vi "visa write read buffer.vi"() -> ()   [LabVIEW 2010]
doc: "This VI will write commands and reads responses from a VISA device."
panel:
  in  "Send Message":bool
  in  "VISA resource name":refnum<visa-resource-name>
  out "Read Buffer":string
  in  "Write Buffer":string="MEAS:AC?"
  in  "stop":bool
  # "Enter message in the Write Buffer\ncontrol and click Send Message to\nsend the message and read the \nresponse from the instrument."
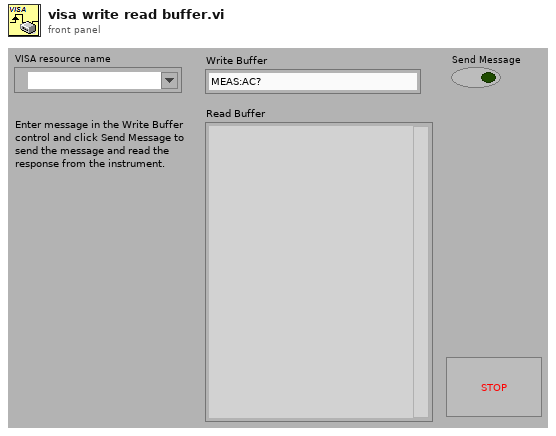
[diagram p1: front panel]
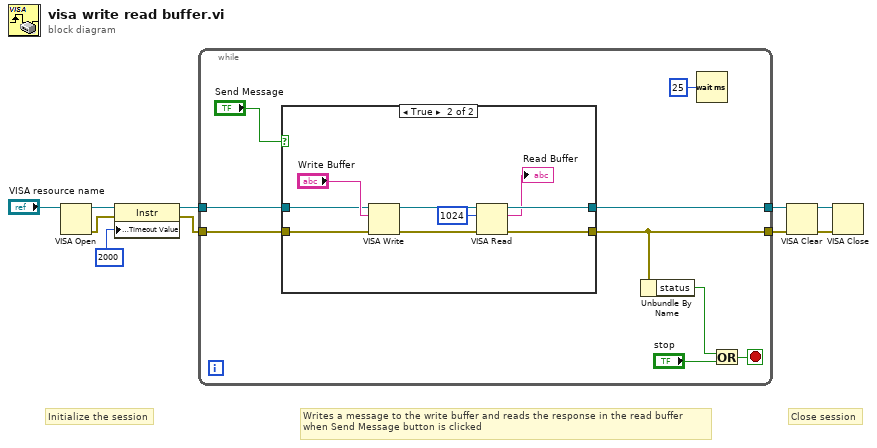
[diagram p0: block diagram]
diagram:
  # "Close session"
  # "Writes a message to the write buffer and reads the response in the read buffer\nwhen Send Message button is clicked"
  # "Initialize the session"
  n1 = VISA Open(VISA resource name="VISA resource name") -> (VISA resource name=w7:refnum<visa-resource-name>, error out=w5:errorcluster)  [unwired: 4 in]
  n2 = property class="Instr"(reference=w7, error in=w5, "General Settings:Timeout Value"=u32 2000) -> (reference out=w6:refnum<visa-resource-name>, error out=w4:errorcluster)
  n3 = while {
    tunnel: w6 -> [w19]
    tunnel: w4 -> [w18]
    tunnel: [w17] -> w10
    tunnel: [w13] -> w2
    stop <- w14 stop-if-true
    n4 = case shown="True" "Send Message" {
      tunnel: w19 -> [w21 w28]
      tunnel: w18 -> [w20 w27]
      tunnel: [w21 w24] -> w17
      tunnel: [w20 w23] -> w13
      frame False {
      }
      frame True {
        n5 = VISA Write(VISA resource name=w28, write buffer="Write Buffer", error in (no error)=w27) -> (VISA resource name out=w25:refnum<visa-resource-name>, error out=w26:errorcluster)  [unwired: 1 out]
        n6 = VISA Read(VISA resource name=w25, byte count=u32 1024, error in (no error)=w26) -> (VISA resource name out=w24:refnum<visa-resource-name>, read buffer=→"Read Buffer":string, error out=w23:errorcluster)  [unwired: 1 out]
      }
    }
    n7 = Unbundle By Name(w13) -> ("status"=w12:bool)
    n8 = Wait (ms)(milliseconds to wait=u32 25) -> ()  [unwired: 1 out]
    n9 = Or(x=w12, y="stop") -> (x .or. y?=w14:bool)
  }
  n10 = VISA Clear(VISA resource name=w10, error in (no error)=w2) -> (VISA resource name out=w3:refnum<visa-resource-name>, error out=w1:errorcluster)
  n11 = VISA Close(VISA resource name=w3, error in (no error)=w1) -> ()  [unwired: 1 out]
